vi "Run_6_of_6_Tests.vi"() -> ()   [LabVIEW 2019]
uses:
  <vilib>/Rock Robotics/WPI/ThirdParty/JAS_Junk/TrajLib/Trajectory_Library.lvlib
panel:
  out "Function Generator":bool
  out "Diff Drive Accel Limiter":bool
  out "String":string
  out "All Tests Finished":bool
  # "FORMAL TRAJECTORY / CONTROL LIBRARY TEST PROCEDURE"
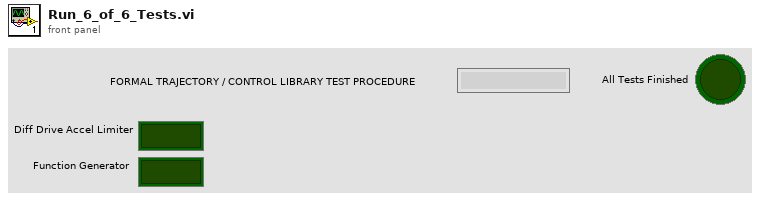
[diagram p1: front panel]
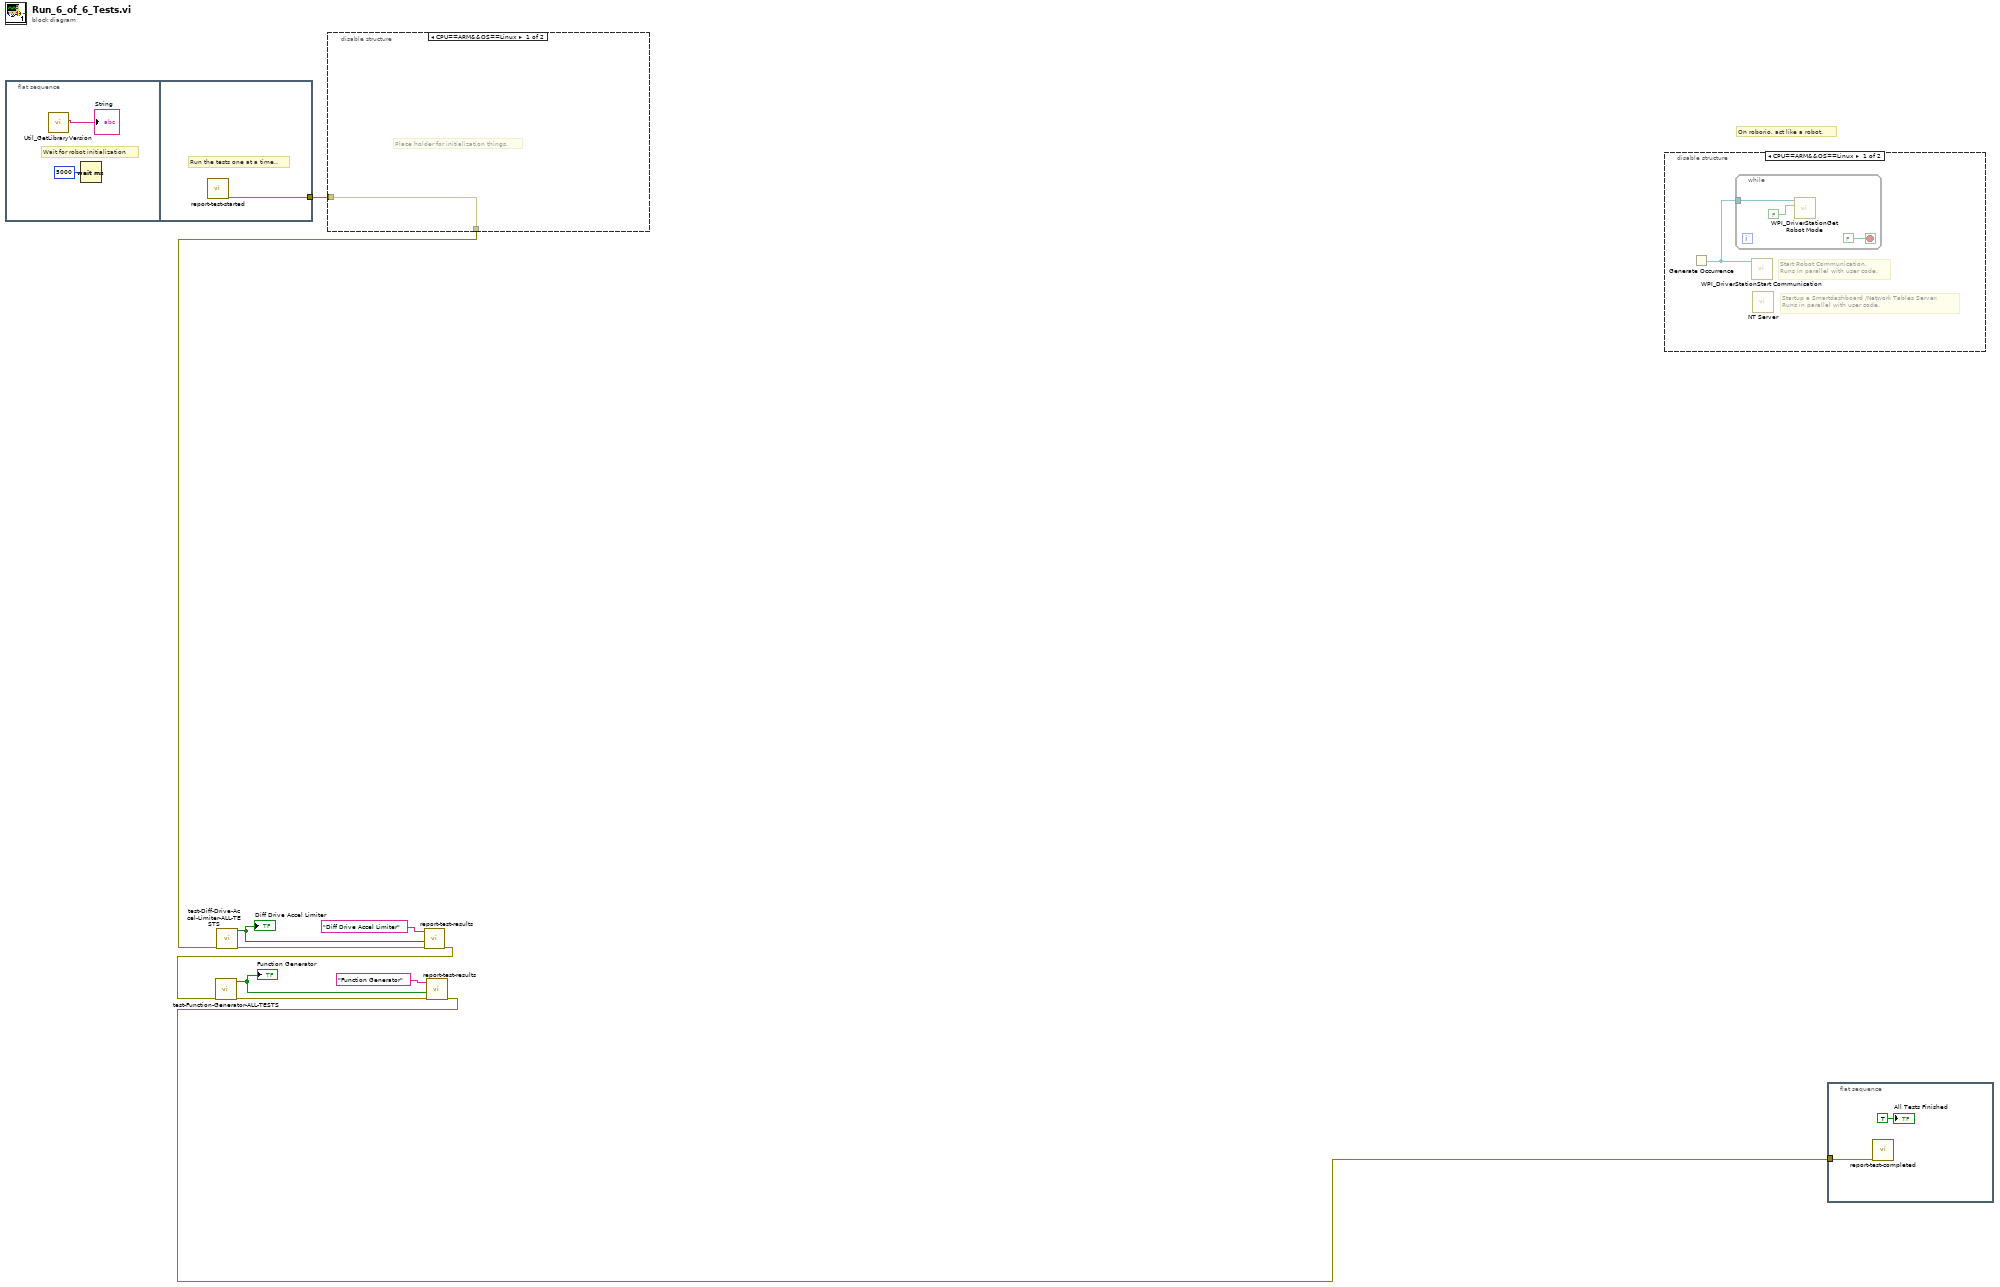
[diagram p0: block diagram]
diagram:
  # "On roborio, act like a robot."
  n1 = flat-sequence {
    tunnel: [w13] -> w10
    frame #0 {
      # "Wait for robot initialization"
      n2 = call <vilib>:"Util_GetLibraryVersion.vi"() -> ("TrajLibVersion"=→"String":string)  [unwired: 11 in]
      n3 = Wait (ms)(milliseconds to wait=u32 5000) -> ()  [unwired: 1 out]
    }
    frame #1 {
      # "Run the tests one at a time.."
      n4 = call "report-test-started.vi"() -> ("error out"=w13:errorcluster)  [unwired: 11 in]
    }
  }
  n5 = disable-structure shown="CPU==ARM&&OS==Linux" {
    disable-tunnel: w10 -> [w14 w15]
    disable-tunnel: [w14 w15] -> w6
    frame condition #0 {
      # "Place holder for initialization things."
    }
    frame condition #1 (active) {
    }
  }
  n6 = call "test-Diff-Drive-Accel-Limiter-ALL-TESTS.vi"("error in (no error)"=w6) -> ("error out"=w8:errorcluster, "All Passed"=w7:bool)  [unwired: 9 in]
  "Diff Drive Accel Limiter" <- w7
  n7 = call "report-test-results.vi"("error in (no error)"=w8, "TestPassed"=w7, "Test Name"="Diff Drive Accel Limiter") -> ("error out"=w2:errorcluster)  [unwired: 8 in]
  n8 = call "test-Function-Generator-ALL-TESTS.vi"("error in (no error)"=w2) -> ("error out"=w4:errorcluster, "All Passed"=w3:bool)  [unwired: 9 in]
  "Function Generator" <- w3
  n9 = call "report-test-results.vi"("error in (no error)"=w4, "TestPassed"=w3, "Test Name"="Function Generator") -> ("error out"=w1:errorcluster)  [unwired: 8 in]
  n10 = disable-structure shown="CPU==ARM&&OS==Linux" {
    frame condition #0 {
      # "Startup a Smartdashboard /Network Tables Server.\nRuns in parallel with user code."
      # "Start Robot Communication.\nRuns in parallel with user code."
      n11 = Generate Occurrence() -> (w16:refnum<k4>)
      n12 = while {
        tunnel: w16 -> [w19]
        stop <- FALSE stop-if-true
        n13 = call <vilib>:"WPI_DriverStationGet Robot Mode.vi"("Finish"=FALSE, "DS Occurrence"=w19) -> ()  [unwired: 10 out]
      }
      n14 = call <vilib>:"WPI_DriverStationStart Communication.vi"("occurrence"=w16) -> ()  [unwired: 2 in, 9 out]
      n15 = call <vilib>:"NT Server.vi"() -> ()  [unwired: 12 in]
    }
    frame condition #1 (active) {
    }
  }
  n16 = flat-sequence {
    tunnel: w1 -> [w20]
    frame #0 {
      n17 = call "report-test-completed.vi"("error in (no error)"=w20) -> ()  [unwired: 10 in, 1 out]
      "All Tests Finished" <- TRUE ("All Tests Finished")
    }
  }
